vi "GetUUTTestdata.vi"(11 "字符串":string) -> (0 "输出簇":T1, 1 "数值":dbl, 2 "数值 2":dbl, 3 "数组":string[](array[string]), 4 "布尔 2":bool, 5 "布尔":bool)   [LabVIEW 2018]
uses:
  Global.vi
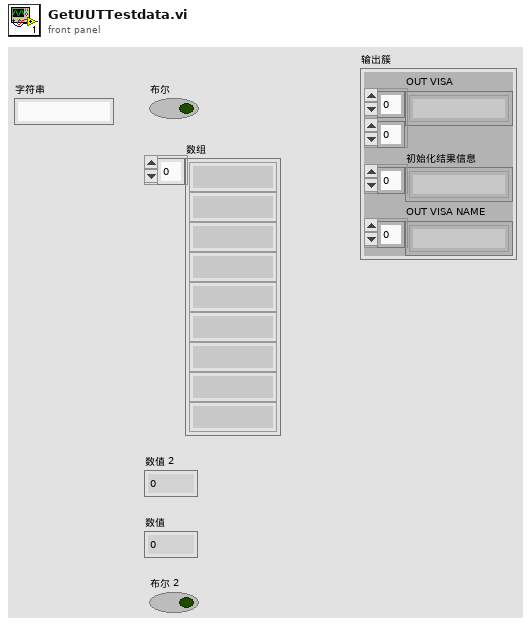
[diagram p1: front panel]
types:
  T1 = cluster{"OUT VISA":string[][], "初始化结果信息":string[], "OUT VISA NAME":string[]}
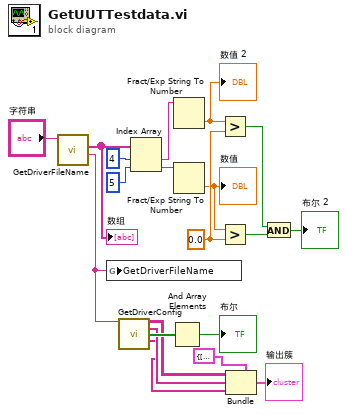
[diagram p0: block diagram]
diagram:
  w16 = 0.0
  n1 = call "GetDriverFileName.vi"("input string"="字符串") -> ("DriverFileName"=w6:string, "数组"=w9:string[])  [unwired: 8 in, 1 out]
  "数组" <- w9
  n2 = global write "Global.vi" "GetDriverFileName"(w6) -> ()
  n3 = call "GetDriverConfig.vi"("TestConfigFileName"=w6) -> ("OUT VISA"=w5:string[][], "初始化结果信息"=w4:string[], "初始化结果"=w7:bool[], "OUT VISA NAME"=w3:string[])  [unwired: 11 in]
  n4 = Index Array(array=w9, index #1=4 ("索引"), index #2=5 ("索引")) -> (element #1=w12:string, element #2=w13:string)
  n5 = And Array Elements(Boolean array=w7) -> (logical AND=→"布尔":bool)
  n6 = Fract/Exp String To Number(string=w12) -> (number=w14:dbl)  [unwired: 3 in, 1 out]
  "数值 2" <- w14
  n7 = Fract/Exp String To Number(string=w13) -> (number=w15:dbl)  [unwired: 3 in, 1 out]
  "数值" <- w15
  n8 = Greater?(x=w14, y=w16) -> (0:w18:bool)
  n9 = Greater?(x=w15, y=w16) -> (0:w17:bool)
  n10 = Bundle(cluster=T1 {"OUT VISA"=[], "初始化结果信息"=[], "OUT VISA NAME"=[]} ("簇"), "OUT VISA"=w5, "初始化结果信息"=w4, "OUT VISA NAME"=w3) -> (→"输出簇":T1)
  n11 = And(x=w18, y=w17) -> (x .and. y?=→"布尔 2":bool)
